vi "TrapProfile_New_DefInitial.vi"(9 "Goal":T2 {"Velocity" format="%16_6e"; "Position" format="%16_6e"}, 11 "Constraints":T1 {"MaxAcceleration" format="%16_6e"; "MaxVelocity" format="%16_6e"}) -> (3 "TRAPEZOID_PROFILE":T3 {"Goal"."Velocity" format="%16_6e"; "Goal"."Position" format="%16_6e"; "Initial"."Velocity" format="%16_6e"; "Initial"."Position" format="%16_6e"; "Constraints"."MaxAcceleration" format="%16_6e"; "Constraints"."MaxVelocity" format="%16_6e"; "EndDecel" format="%16_6e"; "EndFullSpeed" format="%16_6e"; "EndAccel" format="%16_6e"})   [LabVIEW 2019, in "Trajectory_Library.lvlib"]
doc: "Construct a TrapezoidProfile data cluster and performs initial calculations to fill data cluster. A position and velocity of zero are used for as the initial state.\n \nInputs:\n - constraints -- The constraints on the profile, like maximum velocity.\n - goal -- The desired state when the profile is complete.\n\nOutputs:\n - Trapezoid_Profile -- Initialized Trapezoid_Profile data cluster"
uses:
  Trajectory_Library.lvlib
  TRAPEZOID_PROFILE_CONSTRAINT.ctl
  TRAPEZOID_PROFILE_STATE.ctl
  TRAPEZOID_PROFILE.ctl
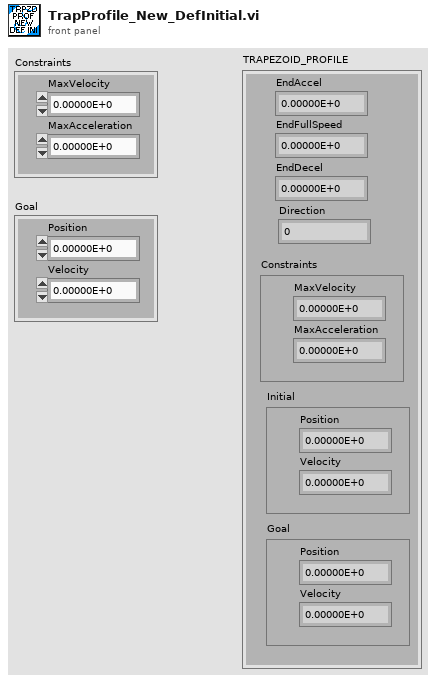
[diagram p1: front panel]
types:
  T1 = typedef "Trajectory_Library.lvlib/TRAPEZOID_PROFILE_CONSTRAINT.ctl" = cluster{"MaxVelocity":dbl, "MaxAcceleration":dbl}
  T2 = typedef "Trajectory_Library.lvlib/TRAPEZOID_PROFILE_STATE.ctl" = cluster{"Position":dbl, "Velocity":dbl}
  T3 = typedef "Trajectory_Library.lvlib/TRAPEZOID_PROFILE.ctl" = cluster{"EndAccel":dbl, "EndFullSpeed":dbl, "EndDecel":dbl, "Direction":i32, "Constraints":T1, "Initial":T2, "Goal":T2}
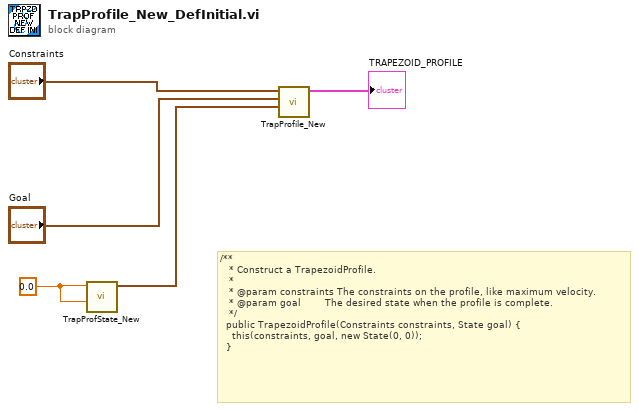
[diagram p0: block diagram]
diagram:
  w1 = 0.0 ("Position")
  # "/**\n   * Construct a TrapezoidProfile.\n   *\n   * @param constraints The constraints on the profile, like maximum velocity.\n   * @param goal        The desired state when the profile is complete.\n   */\n  public TrapezoidProfile(Constraints constraints, State goal) {\n    this(constraints, goal, new State(0, 0));\n  }"
  n1 = call "TrapProfState_New.vi"("Velocity"=w1, "Position"=w1) -> ("TRAPEZOID_PROFILE_STATE"=w2:T2)  [unwired: 9 in]
  n2 = call "TrapProfile_New.vi"("Initial"=w2, "Goal"="Goal", "Constraints"="Constraints") -> ("TRAPEZOID_PROFILE"=→"TRAPEZOID_PROFILE":T3)  [unwired: 8 in]
